vi "Disconnect.vi"(7 "Stage Info":T2={" Current Position"=[-1.0, -12.0, 0.0], "Number of Axis"=3, "ILSID"=1}, 8 "Error In":errorcluster, 11 "Stage-Ctrl":T1={"Console"={"L"=FALSE, "R"=FALSE, "FWD"=FALSE, "BACK"=FALSE}, "Step Width [mm]"=1.0, "Destination [mm]"=[0.0, 0.0], "Move "=FALSE} {"Destination [mm]" format="%_6g"; "Step Width [mm]" min=0.0 format="%_6f"}) -> (0 "Error out":errorcluster)   [LabVIEW 2015]
panel:
  # "X"
  # "Y"
  # "X"
  # "Y"
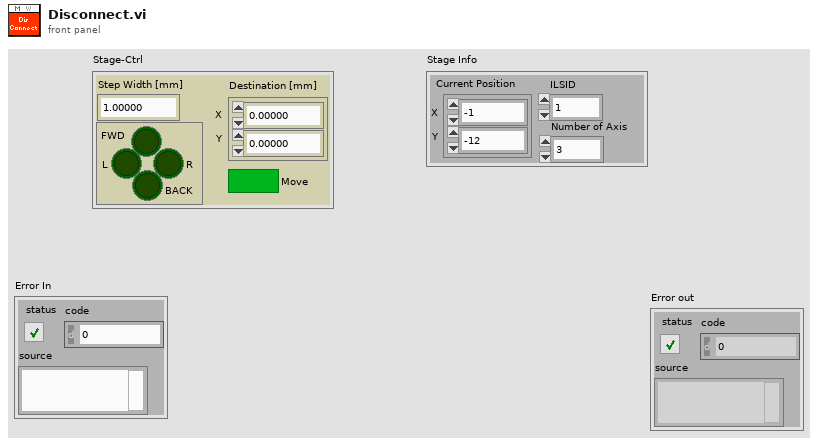
[diagram p1: front panel]
types:
  T1 = cluster{"Console":cluster{"L":bool, "R":bool, "FWD":bool, "BACK":bool}, "Step Width [mm]":dbl, "Destination [mm]":dbl[], "Move ":bool}
  T2 = cluster{" Current Position":dbl[], "Number of Axis":i32, "ILSID":i32}
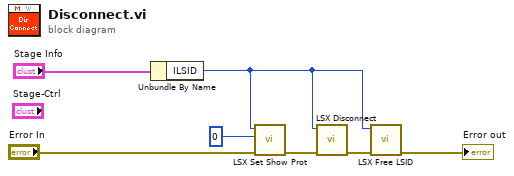
[diagram p0: block diagram]
diagram:
  n1 = Unbundle By Name("Stage Info") -> ("ILSID"=w4:i32)
  n2 = call <userlib>:"LSX Set Show Prot.vi"("error in (no error)"="Error In", "bShowProt"=0, "lLSID"=w4) -> ("error out"=w6:errorcluster)  [unwired: 7 in, 1 out]
  n3 = call <userlib>:"LSX Disconnect.vi"("error in (no error)"=w6, "lLSID"=w4) -> ("error out"=w7:errorcluster)  [unwired: 8 in, 1 out]
  n4 = call <userlib>:"LSX Free LSID.vi"("error in (no error)"=w7, "lLSID"=w4) -> ("error out"=→"Error out":errorcluster)  [unwired: 8 in, 1 out]
